vi "Stop.vi"(8 "error in (no error)":errorcluster, 11 "MQTT_Base in":refnum<class "MQTT_Base.lvclass">) -> (0 "error out":errorcluster, 1 "timed out?":bool, 3 "MQTT_Base out":refnum<class "MQTT_Base.lvclass">)   [LabVIEW 2013, in "MQTT Base.lvlib" / "MQTT_Base.lvclass"]
uses:
  MQTT_Base.lvclass
  MQTT_Base.lvclass/MQTT_Base.ctl
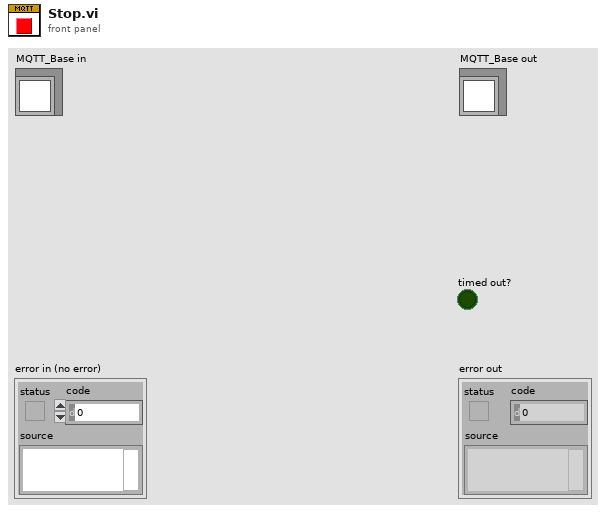
[diagram p1: front panel]
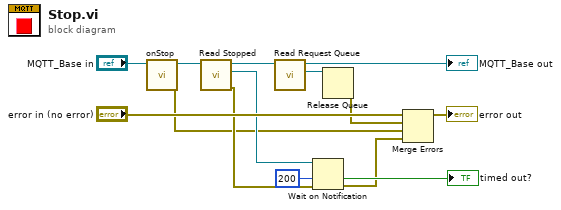
[diagram p0: block diagram]
diagram:
  n1 = call-dynamic "onStop.vi"("MQTT_Base in"="MQTT_Base in") -> ("error out"=w5:errorcluster, "MQTT_Base out"=w2:refnum<class "MQTT_Base.lvclass">)  [unwired: 9 in]
  n2 = call "Read Stopped.vi"("MQTT_Base in"=w2) -> ("error out"=w9:errorcluster, "Stopped"=w10:refnum<notifier>, "MQTT_Base out"=w1:refnum<class "MQTT_Base.lvclass">)  [unwired: 8 in]
  n3 = call "Read Request Queue.vi"("MQTT_Base in"=w1) -> ("Request"=w8:refnum<queue>, "MQTT_Base out"=→"MQTT_Base out":refnum<class "MQTT_Base.lvclass">)  [unwired: 8 in, 1 out]
  n4 = Wait on Notification(notifier=w10, timeout in ms (-1)=200, error in (no error)=w9) -> (timed out?=→"timed out?":bool, error out=w4:errorcluster)  [unwired: 1 in, 2 out]
  n5 = Release Queue(queue=w8) -> (error out=w6:errorcluster)  [unwired: 2 in, 2 out]
  n6 = Merge Errors("error in (no error)", w6, w5, w4) -> (→"error out":errorcluster)
